vi "Math-Arbitrary Distribution.vi"(0 "samples":i32, 5 "Values":dbl[](array[numeric]), 7 "Weights":dbl[](array[numeric])) -> (4 "Array":dbl[](array[numeric]), 15 "error out":errorcluster)   [LabVIEW 2020]
uses:
  LinSpace (x0-dx-npts).vi
  f38435c4-eef0-4a34-a3b8-1e6ce6d15b94.vi
  <vilib>/gmath/statdist.llb/Uniform Random.vi
  <vilib>/gmath/NI_Gmath.lvlib
  <vilib>/Analysis/NI_AALBase.lvlib
panel:
  out "Histogram":T1(graph)
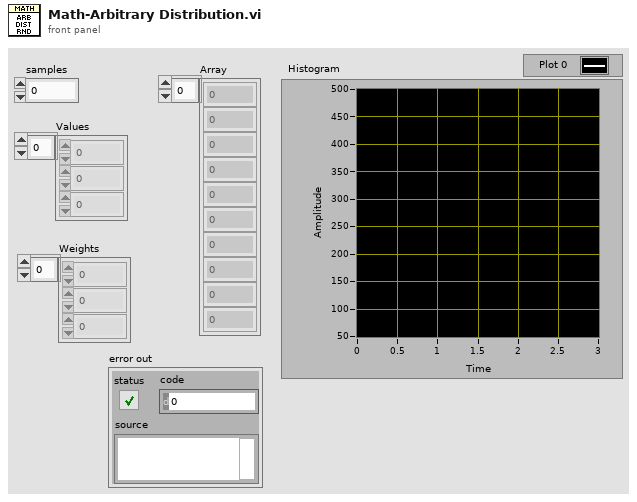
[diagram p1: front panel]
types:
  T1 = cluster{"X Values":dbl[], "Histogram: h(x)":i32[]}
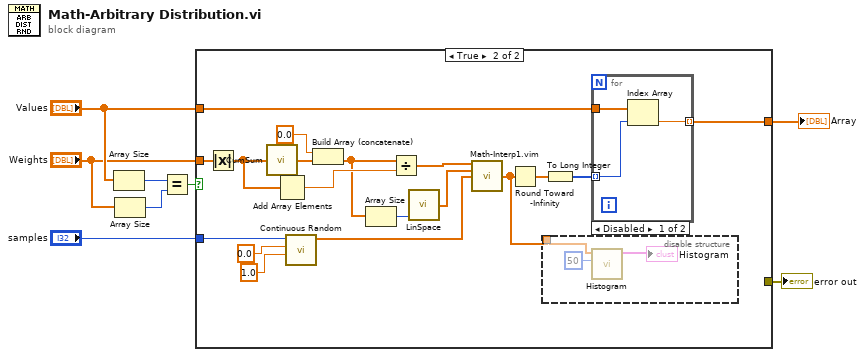
[diagram p0: block diagram]
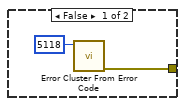
[diagram p2: hidden frame]
diagram:
  n1 = Array Size(array="Values") -> (size(s)=w4:i32)
  n2 = Array Size(array="Weights") -> (size(s)=w3:i32)
  n3 = Equal?(x=w4, y=w3) -> (x = y?=w2:bool)
  n4 = case shown="True" w2 {
    tunnel: "samples" -> [_ w26]
    tunnel: [_ w15] -> w7
    tunnel: "Values" -> [_ w13]
    tunnel: "Weights" -> [_ w12]
    tunnel: [w9 _] -> w1
    frame False {
      n5 = call <vilib>:"Error Cluster From Error Code.vi"("error code (0)"=5118 ("specific error code to clear (0: all)")) -> ("error out"=w9:errorcluster)  [unwired: 8 in]
    }
    frame True {
      n6 = Absolute Value(x=w12) -> (abs(x)=w11:dbl[])
      n7 = call "CumSum.vi"("Array"=w11) -> ("CumSum"=w25:dbl[])
      n8 = Add Array Elements(numeric array=w11) -> (sum=w24:dbl)
      n9 = call-poly <vilib>:"Continuous Random.vi"("xmax"=1.0, "xmin"=0.0, "samples"=w26) -> ("uniform random data"=w20:dbl[])  [unwired: 7 in, 1 out]
      n10 = Build Array (concatenate)(0.0, w25) -> (w18:dbl[])
      n11 = Array Size(array=w18) -> (size(s)=w23:i32)
      n12 = Divide(x=w18, y=w24) -> (x/y=w22:dbl[])
      n13 = call-poly "LinSpace.vi"("npts"=w23) -> ("Array"=w21:dbl[])  [unwired: 3 in, 1 out]
      n14 = call "Math-Interp1.vim"("X"=w22, "Y"=w21, "U"=w20) -> ("V"=w14:dbl[])  [unwired: 12 in]
      n15 = Round Toward -Infinity(1:w14) -> (0:w17:dbl[])
      n16 = disable-structure shown="Disabled" {
        disable-tunnel: w14 -> [w29 _]
        frame Disabled {
          n17 = call <vilib>:"Histogram.vi"("intervals"=50, "X"=w29) -> ("Histogram Graph"=→"Histogram":T1)  [unwired: 6 in, 3 out]
        }
        frame Enabled {
        }
      }
      n18 = To Long Integer(number=w17) -> (32bit integer=w16:i32[])
      n19 = for {
        tunnel: w13 -> [w34]
        tunnel: w16 -> [w33] mode=indexing
        tunnel: [w32] -> w15 mode=indexing
        n20 = Index Array(array=w34, index=w33) -> (element=w32:dbl)
      }
    }
  }
  "Array" <- w7
  "error out" <- w1
